vi "closeRefsMain.vi"(8 "error in (no error)":errorcluster {"code" format="Error %.0f"}, 11 "mainRefs":T1) -> (0 "error out":errorcluster {"code" format="Error %.0f"})   [LabVIEW 2017]
uses:
  Controls/objectRefsMain.ctl
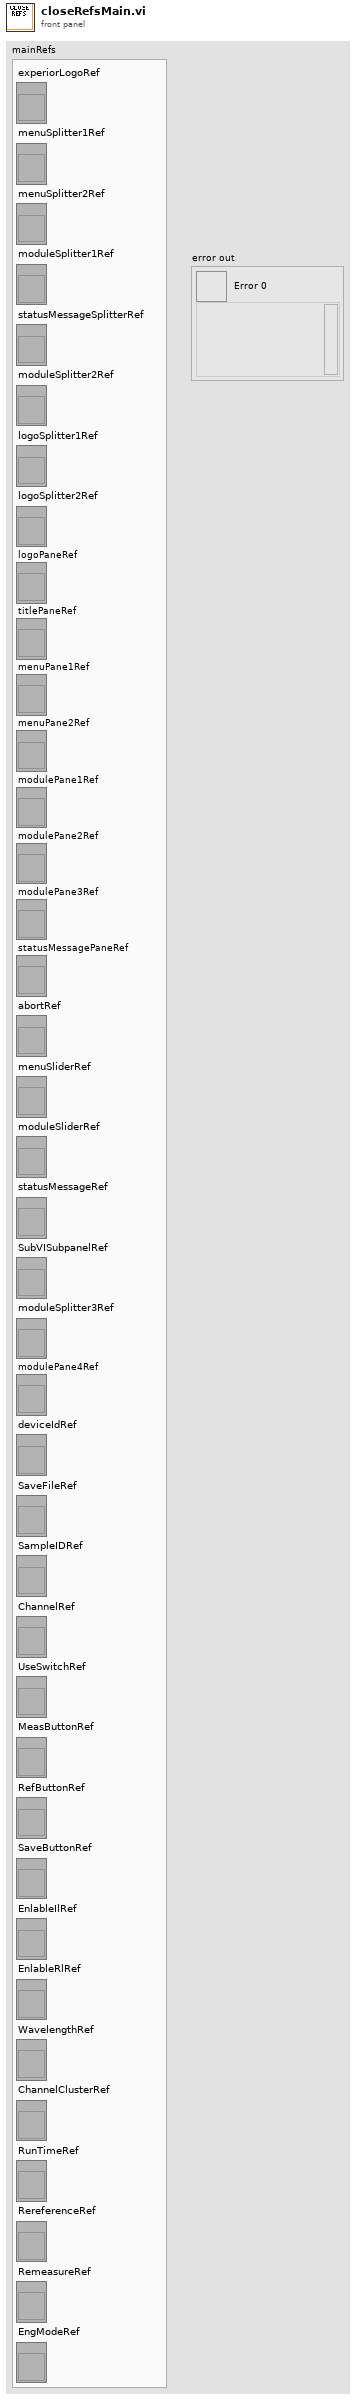
[diagram p1: front panel]
types:
  T1 = typedef "objectRefsMain.ctl" = cluster{"experiorLogoRef":refnum<vi>, "menuSplitter1Ref":refnum<vi>, "menuSplitter2Ref":refnum<vi>, "moduleSplitter1Ref":refnum<vi>, "statusMessageSplitterRef":refnum<vi>, "moduleSplitter2Ref":refnum<vi>, "logoSplitter1Ref":refnum<vi>, "logoSplitter2Ref":refnum<vi>, "logoPaneRef":refnum<vi>, "titlePaneRef":refnum<vi>, "menuPane1Ref":refnum<vi>, "menuPane2Ref":refnum<vi>, "modulePane1Ref":refnum<vi>, "modulePane2Ref":refnum<vi>, "modulePane3Ref":refnum<vi>, "statusMessagePaneRef":refnum<vi>, "abortRef":refnum<vi>, "menuSliderRef":refnum<vi>, "moduleSliderRef":refnum<vi>, "statusMessageRef":refnum<vi>, "SubVISubpanelRef":refnum<vi>, "moduleSplitter3Ref":refnum<vi>, "modulePane4Ref":refnum<vi>, "deviceIdRef":refnum<vi>, "SaveFileRef":refnum<vi>, "SampleIDRef":refnum<vi>, "ChannelRef":refnum<vi>, "UseSwitchRef":refnum<vi>, "MeasButtonRef":refnum<vi>, "RefButtonRef":refnum<vi>, "SaveButtonRef":refnum<vi>, "EnlableIlRef":refnum<vi>, "EnlableRlRef":refnum<vi>, "WavelengthRef":refnum<vi>, "ChannelClusterRef":refnum<vi>, "RunTimeRef":refnum<vi>, "RereferenceRef":refnum<vi>, "RemeasureRef":refnum<vi>, "EngModeRef":refnum<vi>}
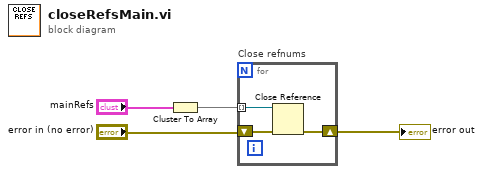
[diagram p0: block diagram]
diagram:
  n1 = Cluster To Array(cluster="mainRefs") -> (array=w4:refnum<vi>[])
  n2 = for "Close refnums" {
    shift-right: [w6] -> w3
    shift-left: "error in (no error)" -> [w7]
    tunnel: w4 -> [w5] mode=indexing
    n3 = Close Reference(reference=w5, error in (no error)=w7) -> (error out=w6:errorcluster)
  }
  "error out" <- w3
